vi "Read Repeat times.vi"(8 "error in (no error)":errorcluster, 11 "Measure Object in":refnum<class "Da Base.lvclass">) -> (0 "error out":errorcluster, 2 "Repeat times":i32=1, 3 "Measure Object out":refnum<class "Da Base.lvclass">)   [LabVIEW 2016, in "Da Base.lvclass"]
uses:
  Da Base.lvclass
  Da Base.lvclass/Da Base.ctl
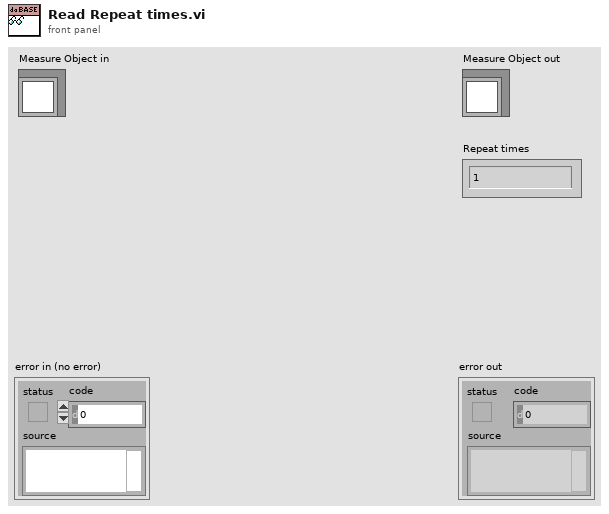
[diagram p1: front panel]
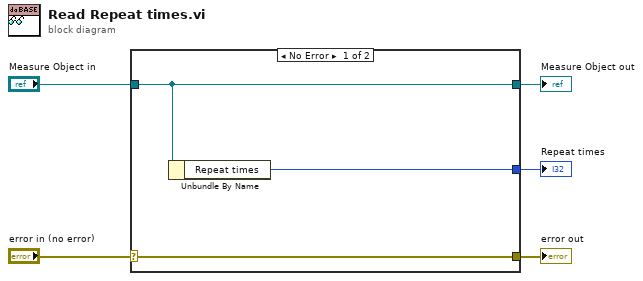
[diagram p0: block diagram]
diagram:
  n1 = case shown="No Error" "error in (no error)" {
    selector: "error in (no error)" -> [w8 w9]
    tunnel: [w8 w9] -> w4
    tunnel: [w7 w10] -> w2
    tunnel: "Measure Object in" -> [w7 w10]
    tunnel: [w6 _] -> w1
    frame No Error {
      n2 = Unbundle By Name(w7) -> ("Repeat times"=w6:i32)
    }
    frame Error {
    }
  }
  "error out" <- w4
  "Measure Object out" <- w2
  "Repeat times" <- w1
